vi "Find and Rename Libraries.vi"(7 "Private Data.Application Ref":refnum<vi>, 8 "error in (no error)":errorcluster, 10 "New TLB Name":string, 11 "Owned Items[]":refnum<vi>[](array[refnum])) -> (0 "error out":errorcluster, 2 "Array 2":string[](array[string]), 3 "Array":string[](array[string]))   [LabVIEW 2018, in "TLB` Springboard.lvlib"]
uses:
  TLB` Springboard.lvlib
  <vilib>/regexp/Match Regular Expression.xnode
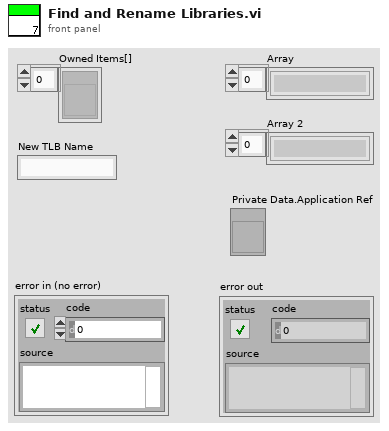
[diagram p1: front panel]
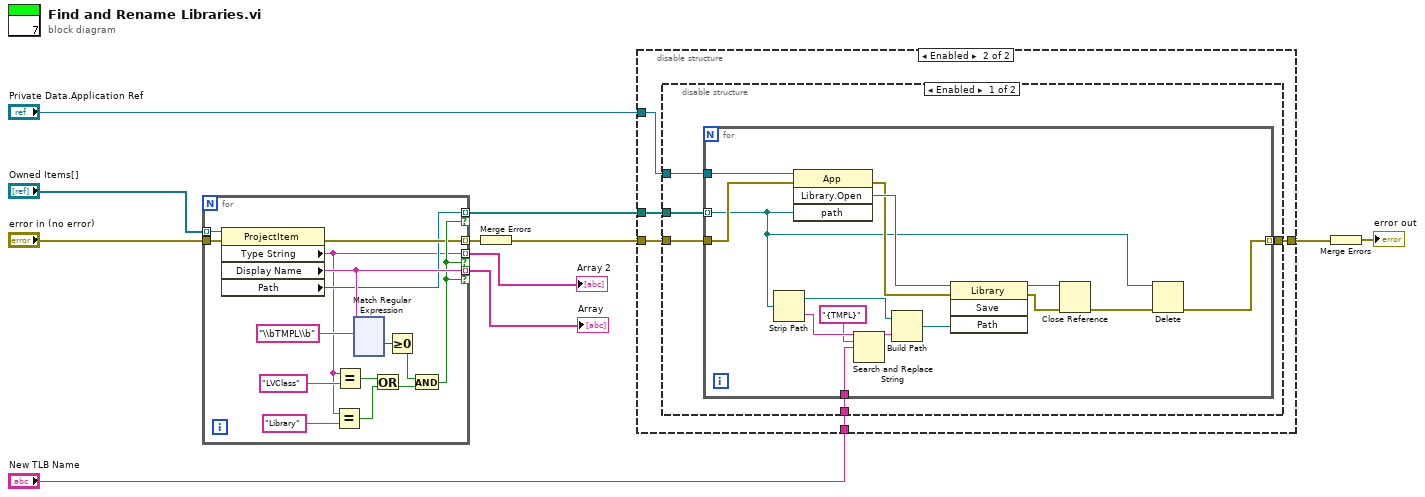
[diagram p0: block diagram]
diagram:
  n1 = for {
    tunnel: "Owned Items[]" -> [w26] mode=indexing
    tunnel: [w13] -> w6 mode=indexing if=w21
    tunnel: [w24] -> w7 mode=indexing if=w21
    tunnel: [w17] -> w1 mode=indexing if=w21
    tunnel: [w20] -> w10 mode=indexing
    tunnel: "error in (no error)" -> [w19]
    n2 = property class="ProjectItem"(reference=w26, error in=w19) -> (error out=w20:errorcluster, "Type String"=w13:string, "Display Name"=w24:string, "Path"=w17:path)  [unwired: 1 out]
    n3 = Equal?(x=w13, y="Library") -> (x = y?=w12:bool)
    n4 = Equal?(x=w13, y="LVClass") -> (x = y?=w15:bool)
    n5 = xnode "Match Regular Expression"("input string"=w24, "regular expression"="\\bTMPL\\b") -> ("offset past match"=w22:i32)  [unwired: 4 in, 4 out]
    n6 = Or(x=w15, y=w12) -> (x .or. y?=w16:bool)
    n7 = Greater Or Equal To 0?(x=w22) -> (x >= 0?=w18:bool)
    n8 = And(x=w18, y=w16) -> (x .and. y?=w21:bool)
  }
  "Array" <- w7
  "Array 2" <- w6
  n9 = Merge Errors(w10) -> (w11:errorcluster)
  n10 = disable-structure shown="Enabled" {
    disable-tunnel: w11 -> [_ w143]
    disable-tunnel: "New TLB Name" -> [_ w141]
    disable-tunnel: [_ w142] -> w4
    disable-tunnel: "Private Data.Application Ref" -> [_ w145]
    disable-tunnel: w1 -> [_ w144]
    frame Disabled {
    }
    frame Enabled {
      n11 = disable-structure shown="Enabled" {
        disable-tunnel: w145 -> [w150 _]
        disable-tunnel: w144 -> [w149 _]
        disable-tunnel: w143 -> [w148 _]
        disable-tunnel: [w147 _] -> w142
        disable-tunnel: w141 -> [w146 _]
        frame Enabled {
          n12 = for {
            tunnel: w150 -> [w165]
            tunnel: w149 -> [w151] mode=indexing
            tunnel: w148 -> [w164]
            tunnel: [w152] -> w147 mode=indexing
            tunnel: w146 -> [w154]
            n13 = Strip Path(path=w151) -> (stripped path=w155:path, name=w158:string)
            n14 = invoke class="App" method="Library.Open"(reference=w165, error in=w164, "path"=w151) -> (error out=w162:errorcluster, "Open Library"=w163:refnum<vi>)  [unwired: 1 in, 2 out]
            n15 = Search and Replace String(input string=w158, search string="{TMPL}", replace string=w154) -> (result string=w156:string)  [unwired: 5 in, 3 out]
            n16 = Build Path(base path=w155, name or relative path=w156) -> (appended path=w153:path)
            n17 = invoke class="Library" method="Save"(reference=w163, error in=w162, "Path"=w153) -> (reference out=w160:refnum<vi>, error out=w161:errorcluster)  [unwired: 1 in, 2 out]
            n18 = Close Reference(reference=w160, error in (no error)=w161) -> (error out=w159:errorcluster)
            n19 = Delete(path (use dialog)=w151, error in=w159) -> (error out=w152:errorcluster)  [unwired: 3 in, 2 out]
          }
        }
        frame Disabled {
        }
      }
    }
  }
  n20 = Merge Errors(w4) -> (→"error out":errorcluster)
